vi "S2C_XML_Globals.vi"() -> ()   [LabVIEW 2015]
panel:
  in  "MeasMeta":cluster{"MetaName":string, "MetaValue":string}[](array[cluster])
  in  "Limits":refnum<k20>
  in  "TestName":string
  in  "XML_Output":path
  out "XML?":bool
  in  "EventData":T1
  in  "Meas(s)":refnum<k20>
  in  "Tests":refnum<k20>
  in  "Meas":refnum<k20>
  in  "Test":refnum<k20>
  out "Event":refnum<k20>
  out "Doc":refnum<k20>
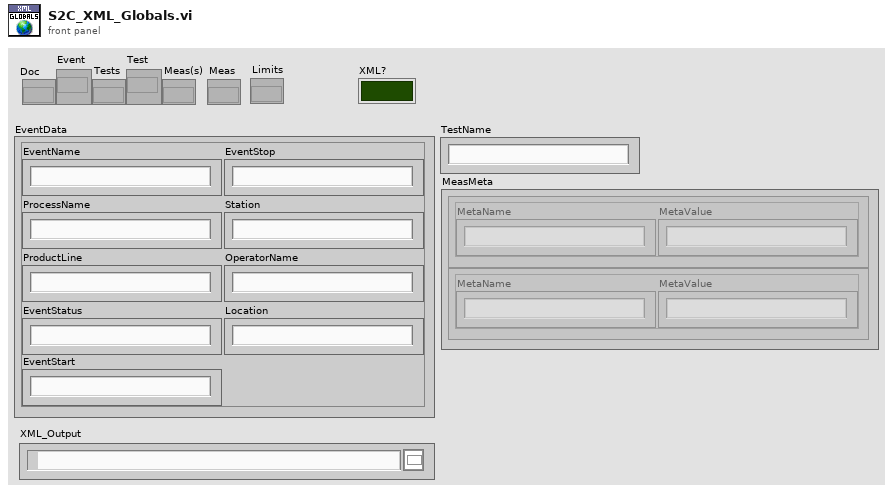
[diagram p1: front panel]
types:
  T1 = cluster{"EventName":string, "ProcessName":string, "ProductLine":string, "EventStatus":string, "EventStart":string, "EventStop":string, "Station":string, "OperatorName":string, "Location":string}
diagram:
